vi "GetTime Stamp.vi"(7 "key description":string, 8 "sections":string[](array[string]), 9 "time stamp":timestamp, 11 "info data":string) -> (0 "sections out":string[](array[string]), 1 "key found?":bool, 2 "value":timestamp, 3 "info data out":string)   [LabVIEW 2020, in "infolib.lvlib"]
doc: "Add a new numeric key to Info Data string. If section exists in Info Data string, inserts key into this section."
uses:
  infolib.lvlib
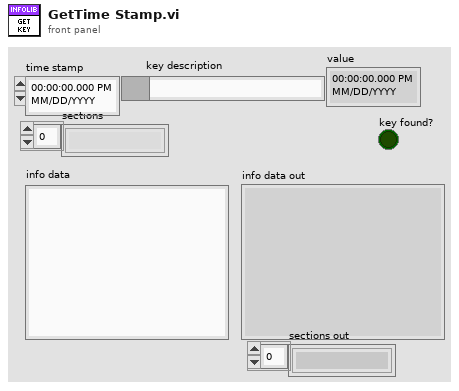
[diagram p1: front panel]
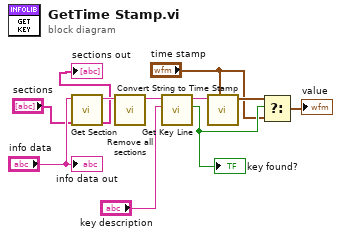
[diagram p0: block diagram]
diagram:
  n1 = call "Get Section.vi"("sections"="sections", "info data"="info data") -> ("sections out"=→"sections out":string[], "section part"=w11:string)  [unwired: 7 in, 1 out]
  n2 = call "Remove all sections.vi"("info data"=w11) -> ("info data out"=w10:string)  [unwired: 10 in]
  n3 = call "Get Key Line.vi"("key description"="key description", "info data"=w10) -> ("key found?"=w3:bool, "key value"=w7:string)  [unwired: 8 in]
  "key found?" <- w3
  n4 = call "Convert String to Time Stamp.vi"("default value of time stamp"="time stamp", "string"=w7) -> ("time stamp out"=w4:timestamp)  [unwired: 9 in]
  n5 = Select(t=w4, s=w3, f="time stamp") -> (s? t:f=→"value":timestamp)
  "info data out" <- "info data"
